vi "testGuess-2_PPM.vi"(8 "error in (no error)":errorcluster, 11 "TestCase in":refnum<class "ScoringTestCase.lvclass">) -> (0 "error out":errorcluster, 3 "TestCase out":refnum<class "ScoringTestCase.lvclass">)   [LabVIEW 2017, in "ScoringTestCase.lvclass"]
uses:
  ScoringTestCase.lvclass
  <vilib>/addons/_JKI Toolkits/VI Tester/TestCase.llb/TestCase.lvclass
  C:/Program Files (x86)/National Instruments/LabVIEW 2017/vi.lib/addons/_JKI Toolkits/VI Tester/TestCase.llb/TestCase.lvclass
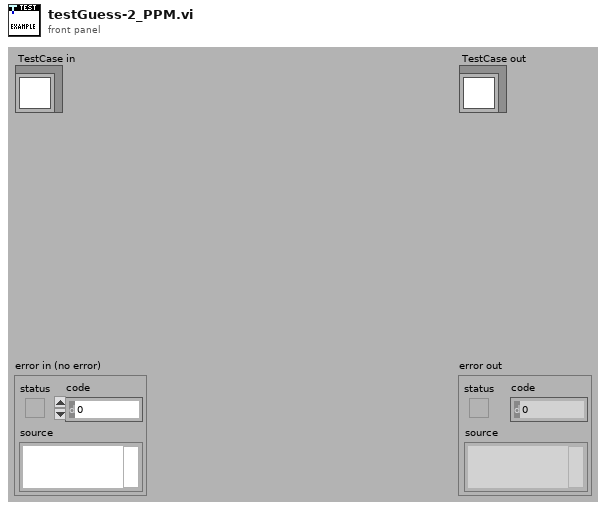
[diagram p1: front panel]
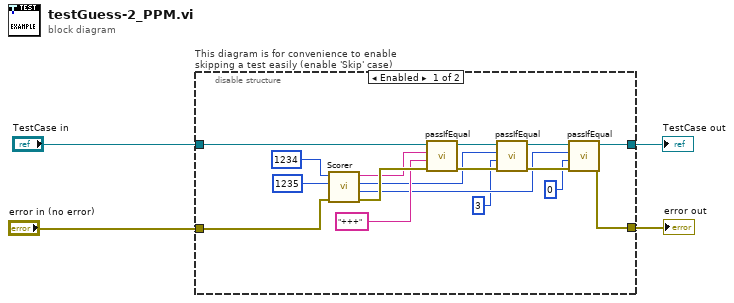
[diagram p0: block diagram]
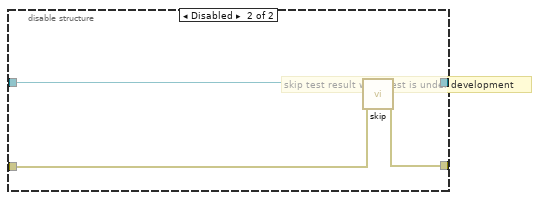
[diagram p2: hidden frame]
diagram:
  n1 = disable-structure "This diagram is for convenience to enable skipping a test easily (enable 'Skip' case)" shown="Enabled" {
    disable-tunnel: "TestCase in" -> [w21 w25]
    disable-tunnel: [w9 w23] -> w1
    disable-tunnel: [w11 w24] -> w3
    disable-tunnel: "error in (no error)" -> [w19 w22]
    frame Enabled {
      n2 = call "Scorer.vi"("error in (no error)"=w19, "Guess"=1235, "Answer"=1234) -> ("error out"=w18:errorcluster, "Minuses"=w7:i32, "Pluses"=w8:i32, "Result"=w17:string)  [unwired: 5 in]
      n3 = call-dynamic "passIfEqual.vi"("error in (no error)"=w18, "y"="+++", "x"=w17, "TestCase in"=w21) -> ("error out"=w20:errorcluster, "TestCase out"=w12:refnum<class "ScoringTestCase.lvclass">)  [unwired: 6 in]
      n4 = call-dynamic "passIfEqual.vi"("error in (no error)"=w20, "y"=3, "x"=w8, "TestCase in"=w12) -> ("error out"=w13:errorcluster, "TestCase out"=w10:refnum<class "ScoringTestCase.lvclass">)  [unwired: 6 in]
      n5 = call-dynamic "passIfEqual.vi"("error in (no error)"=w13, "y"=0, "x"=w7, "TestCase in"=w10) -> ("error out"=w11:errorcluster, "TestCase out"=w9:refnum<class "ScoringTestCase.lvclass">)  [unwired: 6 in]
    }
    frame Disabled {
      # "skip test result while test is under development"
      n6 = call <vilib>:"skip.vi"("error in (no error)"=w22, "TestCase in"=w25) -> ("error out"=w24:errorcluster, "TestCase out"=w23:refnum<class "ScoringTestCase.lvclass">)  [unwired: 8 in]
    }
  }
  "error out" <- w3
  "TestCase out" <- w1
